vi "Create Attribute (Data Item).vi"(10 "Value":refnum<class "Data Item.lvclass">, 11 "Name":string) -> (3 "Attribute":refnum<class "Attribute.lvclass">)   [LabVIEW 2023, in "VILab.lvlib" / "Attribute.lvclass"]
uses:
  Attribute.lvclass
  Data Item/Data Item.lvclass
  Attribute.lvclass/Attribute.ctl
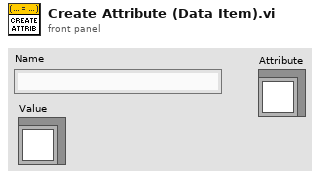
[diagram p1: front panel]
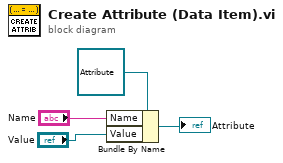
[diagram p0: block diagram]
diagram:
  n1 = Bundle By Name(cluster=refnum<class "Attribute.lvclass"> refnum ("VILab.lvlib:Attribute.lvclass"), "Name"="Name", "Value"="Value") -> (→"Attribute":refnum<class "Attribute.lvclass">)
